vi "Read Focus region centers.vi"(8 "error in (no error)":errorcluster, 11 "Update Focus Msg in":refnum<class "Update Focus Msg.lvclass">) -> (0 "error out":errorcluster, 2 "Focus region centers":dbl[](array[numeric]), 3 "Update Focus Msg out":refnum<class "Update Focus Msg.lvclass">)   [LabVIEW 2016, in "Update Focus Msg.lvclass"]
uses:
  Update Focus Msg.lvclass
  Update Focus Msg.lvclass/Update Focus Msg.ctl
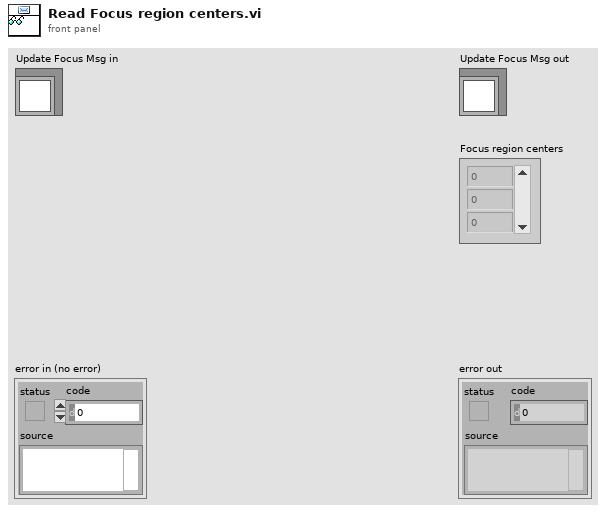
[diagram p1: front panel]
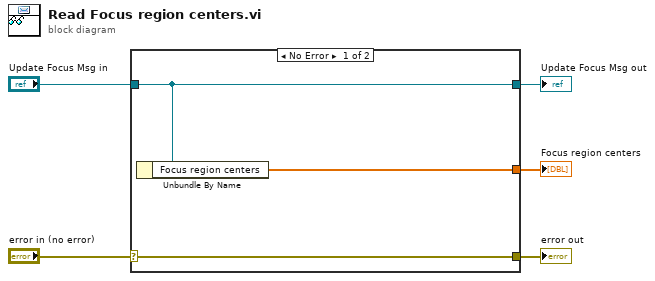
[diagram p0: block diagram]
diagram:
  n1 = case shown="No Error" "error in (no error)" {
    selector: "error in (no error)" -> [w8 w9]
    tunnel: [w8 w9] -> w4
    tunnel: [w7 w10] -> w2
    tunnel: "Update Focus Msg in" -> [w7 w10]
    tunnel: [w6 _] -> w1
    frame No Error {
      n2 = Unbundle By Name(w7) -> ("Focus region centers"=w6:dbl[])
    }
    frame Error {
    }
  }
  "error out" <- w4
  "Update Focus Msg out" <- w2
  "Focus region centers" <- w1
